vi "UpdateImage.vi"(0 "reference in":refnum<class "LcPictureBox.lvclass">, 5 "Error In":errorcluster) -> (14 "reference out":refnum<class "LcPictureBox.lvclass">, 15 "ImageUsed":refnum<k24>, 16 "DrawingTime(ms)":u32, 19 "Error Out":errorcluster)   [LabVIEW 2020, in "LcPictureBox.lvclass"]
uses:
  LcPictureBox.lvclass
  System.Drawing
  System.Windows.Forms
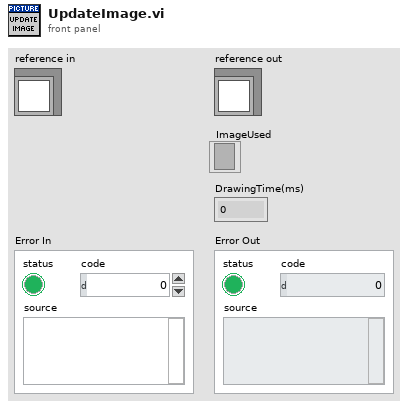
[diagram p1: front panel]
types:
  T1 = typedef "LcPictureBox.lvclass/ObjectAttributes.ctl" = cluster{"PictureBox":refnum<k24>, "ImageSize":cluster{"Width":i32, "Height":i32}, "PenMemory":map{cluster{"Alpha(100%)":dbl, "Color(Black)":u32, "Pen(Width=1, Solid)":T2}, refnum<k24>}, "GraphicsRef":refnum<k24>, "BrushMemory":map{cluster{"Alpha(100%)":dbl, "Color(Black)":u32}, refnum<k24>}, "Images":refnum<k24>[], "ImageIndex":i32, "BgColor(None)":u32, "LoadedImages":map{string, cluster{"ImageOut":refnum<k24>, "ImageSize":cluster{"Width":i32, "Height":i32}}}, "ColorsMemory":map{cluster{"Alpha(100%)":dbl, "Color(Black)":u32}, refnum<k24>}, "CacheSize":i32, "PictureBoxActiveXReference":refnum<vi>, "Scale":sgl, "Offset":cluster{"x":sgl, "y":sgl}, "zoom_center":cluster{"X":i32, "Y":i32}, "ImagesCreated":refnum<k24>[]}
  T2 = typedef "LcPictureBox.lvclass/Pen.ctl" = cluster{"Width":u16, "Style":enum32{"Solid", "Dash", "Dot", "DashDot", "DashDotDot"}}
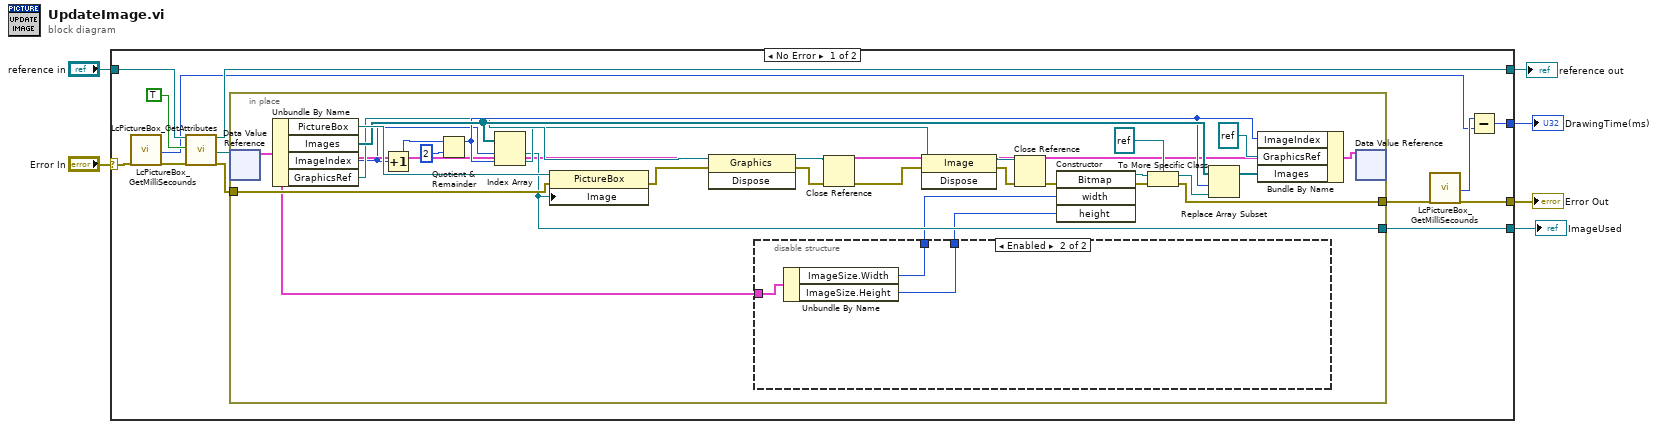
[diagram p0: block diagram]
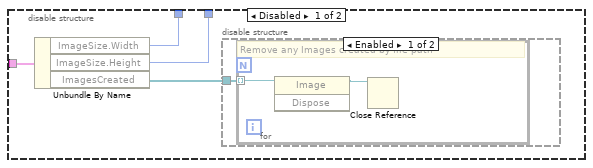
[diagram p2: hidden frame]
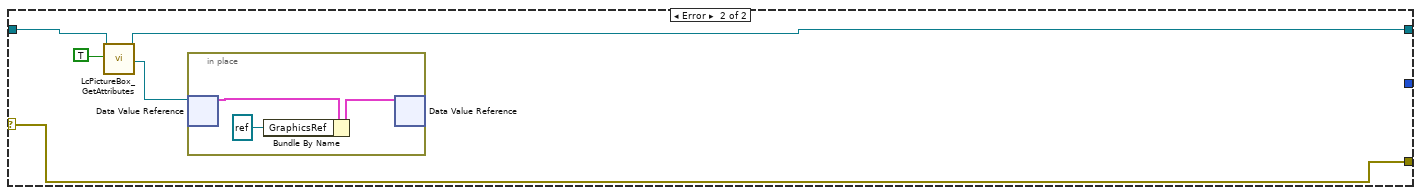
[diagram p4: hidden frame]
diagram:
  n1 = case shown="No Error" "Error In" {
    selector: "Error In" -> [w15 w58]
    tunnel: [w13 w58] -> w5
    tunnel: [w19 w62] -> w3
    tunnel: "reference in" -> [w14 w59]
    tunnel: [w9 _] -> w2
    tunnel: [w8 _] -> w1
    frame No Error {
      n2 = call "LcPictureBox_GetMilliSecounds.vi"("error in (no error)"=w15) -> ("msValue"=w10:u32, "error out"=w11:errorcluster)  [unwired: 17 in]
      n3 = call "LcPictureBox_GetAttributes.vi"("reference in"=w14, "OnlyGetDvrReference(False)"=TRUE, "error in (no error)"=w11) -> ("reference out"=w19:refnum<class "LcPictureBox.lvclass">, "DataRef"=w18:refnum<data-value>, "error out"=w16:errorcluster)  [unwired: 13 in, 1 out]
      n4 = in-place {
        in-place-border: w16 -> [w46]
        in-place-border: [w35] -> w7
        in-place-border: [w27] -> w8
        n5 = in-place-dvr #1(w18) -> (w24:T1)  [unwired: 1 out]
        n6 = Unbundle By Name(w24) -> ("PictureBox"=w47:refnum<k24>, "Images"=w39:refnum<k24>[], "ImageIndex"=w20:i32, "GraphicsRef"=w33:refnum<k24>)
        n7 = Increment(x=w20) -> (x+1=w26:i32)
        n8 = Quotient & Remainder(x=w26, y=2) -> (x-y*floor(x/y)=w38:i32)  [unwired: 1 out]
        n9 = Index Array(array=w39, index #1=w20, index #2=w38) -> (element #1=w27:refnum<k24>, element #2=w29:refnum<k24>)
        n10 = property class="PictureBox"(reference=w47, error in=w46, "Image"=w27) -> (error out=w22:errorcluster)  [unwired: 1 out]
        n11 = invoke class="Graphics" method="Dispose"(reference=w33, error in=w22) -> (reference out=w32:refnum<k24>, error out=w31:errorcluster)  [unwired: 1 in, 1 out]
        n12 = disable-structure shown="Enabled" {
          disable-tunnel: w24 -> [w51 w57]
          disable-tunnel: [w50 w55] -> w23
          disable-tunnel: [w49 w56] -> w21
          frame Disabled {
            n13 = Unbundle By Name(w51) -> ("ImageSize.Width"=w49:i32, "ImageSize.Height"=w50:i32, "ImagesCreated"=w48:refnum<k24>[])
            n14 = disable-structure shown="Enabled" {
              disable-tunnel: w48 -> [w52 _]
              frame Enabled {
                n15 = for {
                  tunnel: w52 -> [w53] mode=indexing
                  # "Remove any Images created by file path"
                  n16 = invoke class="Image" method="Dispose"(reference=w53) -> (reference out=w54:refnum<k24>)  [unwired: 2 in, 2 out]
                  n17 = Close Reference(reference=w54) -> ()  [unwired: 1 in, 1 out]
                }
              }
              frame Disabled {
              }
            }
          }
          frame Enabled {
            n18 = Unbundle By Name(w57) -> ("ImageSize.Width"=w56:i32, "ImageSize.Height"=w55:i32)
          }
        }
        n19 = Close Reference(reference=w32, error in (no error)=w31) -> (error out=w25:errorcluster)
        n20 = invoke class="Image" method="Dispose"(reference=w29, error in=w25) -> (reference out=w28:refnum<k24>, error out=w30:errorcluster)  [unwired: 1 in, 1 out]
        n21 = Close Reference(reference=w28, error in (no error)=w30) -> (error out=w34:errorcluster)
        n22 = constructor class="Bitmap"(error in=w34, "width"=w21, "height"=w23) -> (reference out=w41:refnum<k24>, error out=w40:errorcluster)  [unwired: 2 in, 3 out]
        n23 = To More Specific Class(target class=refnum<k24> refnum, reference=w41, error in=w40) -> (specific class reference=w36:refnum<k24>, error out=w35:errorcluster)
        n24 = Replace Array Subset(array=w39, new element=w36, index=w38) -> (w37:refnum<k24>[])
        n25 = Bundle By Name(cluster=w24, "ImageIndex"=w38, "GraphicsRef"=refnum<k24> refnum, "Images"=w37) -> (w45:T1)
        n26 = in-place-dvr #1(w45) -> ()  [unwired: 2 out]
      }
      n27 = call "LcPictureBox_GetMilliSecounds.vi"("error in (no error)"=w7) -> ("msValue"=w12:u32, "error out"=w13:errorcluster)  [unwired: 17 in]
      n28 = Subtract(x=w12, y=w10) -> (x-y=w9:u32)
    }
    frame Error {
      n29 = call "LcPictureBox_GetAttributes.vi"("reference in"=w59, "OnlyGetDvrReference(False)"=TRUE) -> ("reference out"=w62:refnum<class "LcPictureBox.lvclass">, "DataRef"=w61:refnum<data-value>)  [unwired: 14 in, 2 out]
      n30 = in-place {
        n31 = in-place-dvr #2(w61) -> (w63:T1)  [unwired: 1 out]
        n32 = Bundle By Name(cluster=w63, "GraphicsRef"=refnum<k24> refnum) -> (w65:T1)
        n33 = in-place-dvr #2(w65) -> ()  [unwired: 2 out]
      }
    }
  }
  "Error Out" <- w5
  "reference out" <- w3
  "DrawingTime(ms)" <- w2
  "ImageUsed" <- w1
